vi "RuptureAnalysis.vi"(10 "Tracenames":string[](array[string])) -> ()   [LabVIEW 2018]
uses:
  <vilib>/Utility/file.llb/Read From Spreadsheet File (string).vi
  <vilib>/Utility/file.llb/Write To Spreadsheet File (string).vi
  <vilib>/Analysis/NI_AALPro.lvlib
panel:
  out "Fit result":string[][](array[string])
  in  "stop":bool
  out "Rupture analysis":cluster{dbl[], "Best Linear Fit":dbl[]}[](graph)
  out "Distribution":dynamicdata(graph) caption="Histogram"
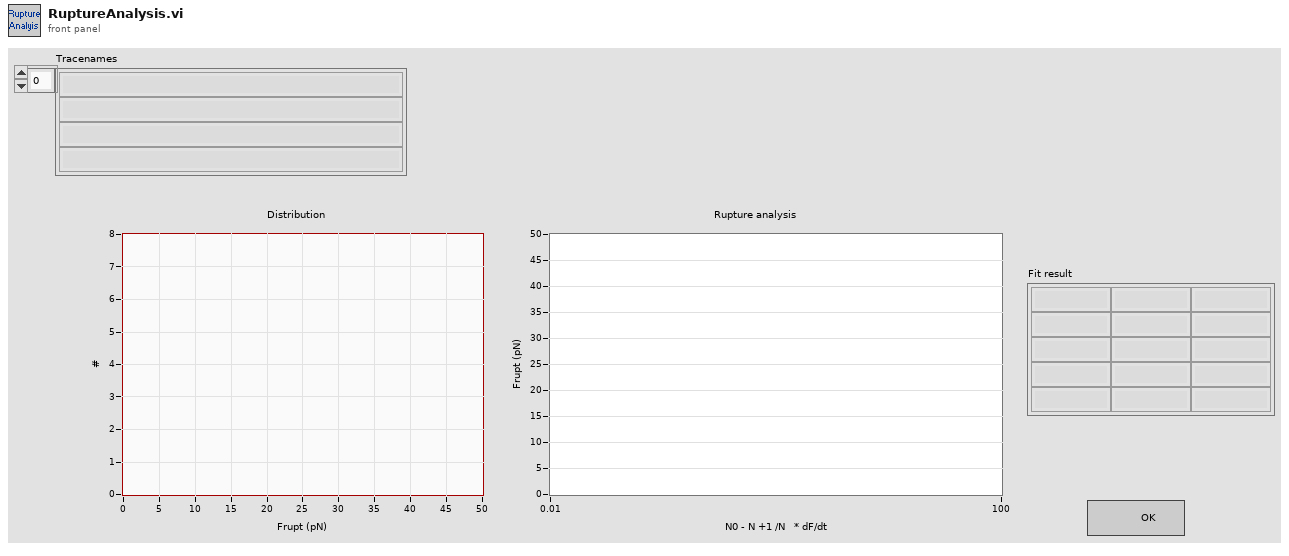
[diagram p1: front panel]
types:
  T1 = enum16{"Init", "Reset", "Update var pars", "Update SE's", "Get", "Save to file", "Read from file"}
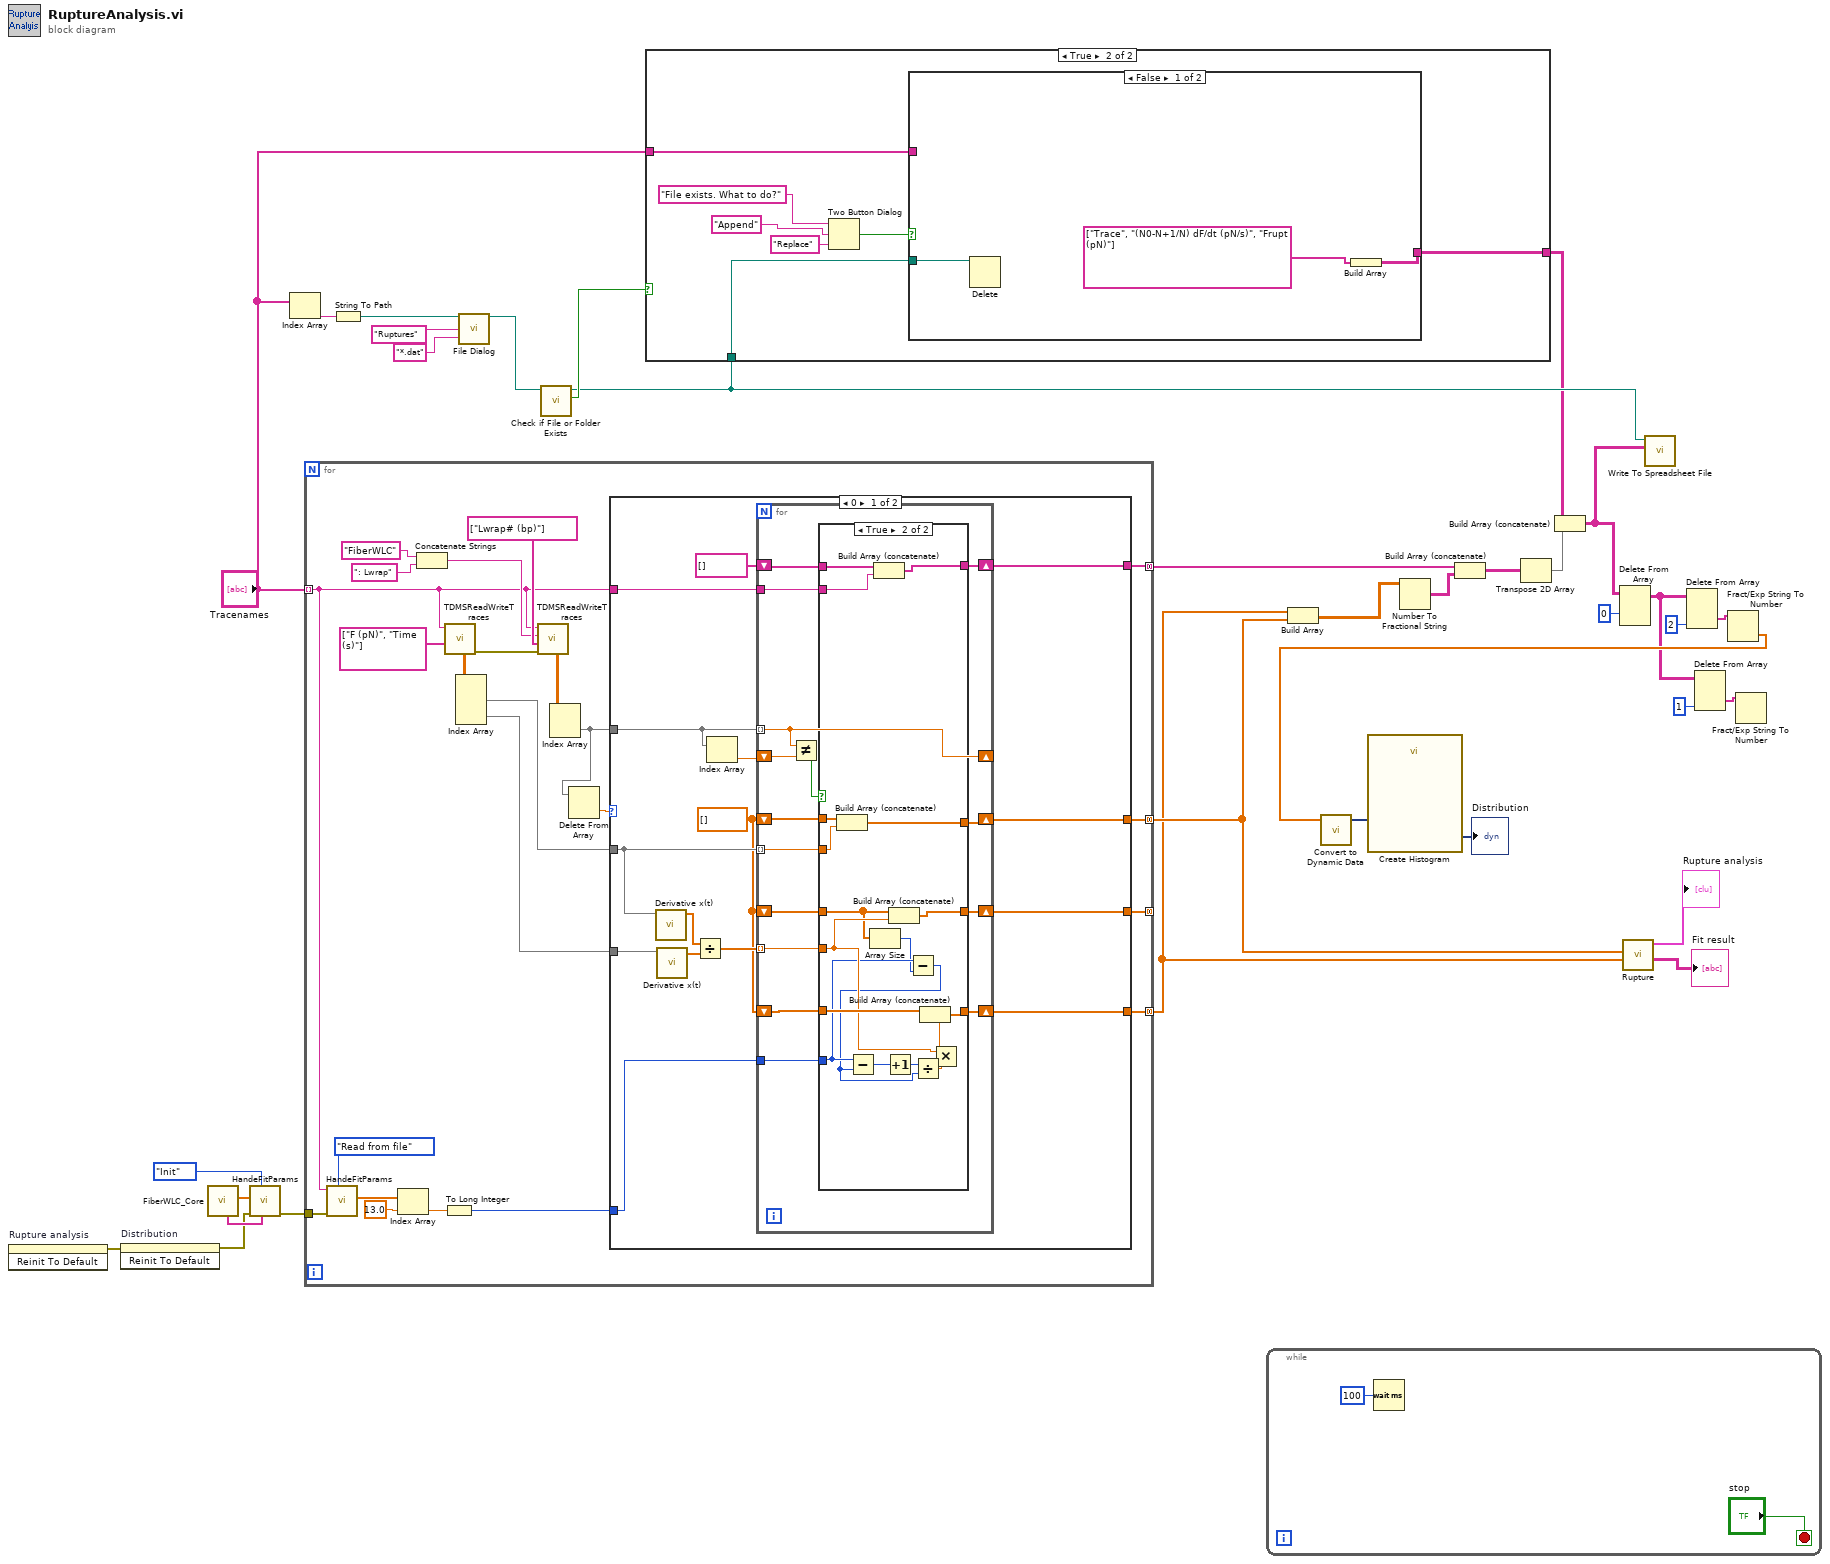
[diagram p0: block diagram]
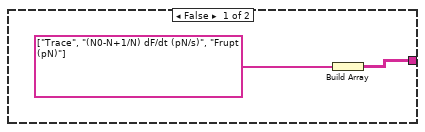
[diagram p2: hidden frame]
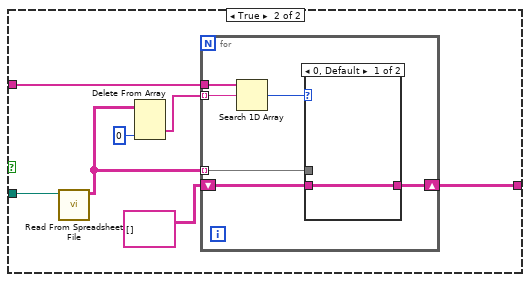
[diagram p3: hidden frame]
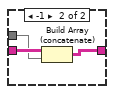
[diagram p4: hidden frame]
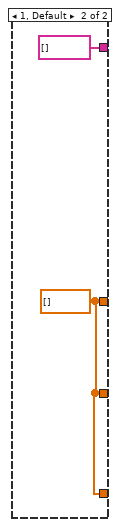
[diagram p6: hidden frame]
diagram:
  n1 = invoke on="Rupture analysis" class="XYGraph (strict)" method="Reinit To Default"() -> (error out=w6:errorcluster)  [unwired: 3 in, 2 out]
  n2 = invoke on="Distribution" class="WFGraph (strict)" method="Reinit To Default"(error in=w6) -> (error out=w7:errorcluster)  [unwired: 2 in, 2 out]
  n3 = call "FiberWLC_Core.vi"() -> ("default params"=w31:dbl[], "default parnames"=w32:string[])  [unwired: 8 in, 2 out]
  n4 = call "HandeFitParams.vi"("Par names"=w32, "task"=T1."Init", "error in (no error)"=w7, "Vars in"=w31) -> ("error out"=w29:errorcluster)  [unwired: 4 in, 3 out]
  n5 = Index Array(array="Tracenames") -> (element=w21:string)  [unwired: 1 in]
  n6 = for {
    tunnel: "Tracenames" -> [w36] mode=indexing
    tunnel: [w49] -> w4 mode=concatenating
    tunnel: [w46] -> _ mode=concatenating
    tunnel: w29 -> [w40]
    tunnel: [w38] -> w3 mode=concatenating
    tunnel: [w35] -> w22 mode=concatenating
    n7 = call "HandeFitParams.vi"("task"=T1."Read from file", "error in (no error)"=w40, "tracename in"=w36) -> ("Vars out"=w42:dbl[])  [unwired: 5 in, 3 out]
    n8 = Index Array(array=w42, index=13.0 ("element")) -> (element=w39:dbl)
    n9 = Concatenate Strings("FiberWLC" ("group name"), ": Lwrap" ("string")) -> (w56:string)
    n10 = To Long Integer(number=w39) -> (32bit integer=w37:i32)
    n11 = call "TDMSReadWriteTraces.vi"("Channels in"=string[] ["F (pN)", "Time (s)"] ("channel name(s) in"), "tracename"=w36) -> ("error out"=w52:errorcluster, "Data out"=w50:dbl[][])  [unwired: 4 in, 4 out]
    n12 = Index Array(array=w50) -> (element #1=w48:dbl[], element #2=w47:dbl[])  [unwired: 4 in]
    n13 = call "TDMSReadWriteTraces.vi"("error in (no error)"=w52, "Channels in"=string[] ["Lwrap# (bp)"], "group name"=w56, "tracename"=w36) -> ("Data out"=w53:dbl[][])  [unwired: 2 in, 5 out]
    n14 = Index Array(array=w53) -> (element=w45:dbl[])  [unwired: 2 in]
    n15 = Delete From Array(array=w45) -> (deleted portion=w44:dbl)  [unwired: 2 in, 1 out]
    n16 = case shown="0" w44 {
      tunnel: [w71 w111] -> w49
      tunnel: w48 -> [w65 _]
      tunnel: w47 -> [w70 _]
      tunnel: [w66 w111] -> w46
      tunnel: w45 -> [w64 _]
      tunnel: w37 -> [w63 _]
      tunnel: [w61 w111] -> w38
      tunnel: w36 -> [w60 _]
      tunnel: [w59 string[] []] -> w35
      frame 0 {
        w62 = dbl[] []
        n17 = call <vilib>:"Derivative x(t).vi"("X"=w65) -> ("dX/dt"=w69:dbl[])  [unwired: 9 in, 1 out]
        n18 = call <vilib>:"Derivative x(t).vi"("X"=w70) -> ("dX/dt"=w68:dbl[])  [unwired: 9 in, 1 out]
        n19 = Divide(x=w69, y=w68) -> (x/y=w67:dbl[])
        n20 = Index Array(array=w64) -> (element=w72:dbl)  [unwired: 1 in]
        n21 = for {
          shift-right: [w86] -> _
          shift-left: w72 -> [w87]
          tunnel: w64 -> [w86] mode=indexing
          tunnel: w65 -> [w83] mode=indexing
          shift-right: [w82] -> w71
          shift-left: w62 -> [w84]
          shift-right: [w81] -> w66
          shift-left: w62 -> [w80]
          tunnel: w67 -> [w79] mode=indexing
          tunnel: w63 -> [w78]
          shift-right: [w77] -> w61
          shift-left: w62 -> [w76]
          shift-right: [w73] -> w59
          shift-left: string[] [] -> [w74]
          tunnel: w60 -> [w75]
          n22 = Not Equal?(x=w86, y=w87) -> (x != y?=w85:bool)
          n23 = case shown="True" w85 {
            tunnel: w84 -> [w91 w109]
            tunnel: w83 -> [_ w108]
            tunnel: [w91 w107] -> w82
            tunnel: [w90 w106] -> w81
            tunnel: w80 -> [w90 w96]
            tunnel: w79 -> [_ w99]
            tunnel: w78 -> [_ w98]
            tunnel: [w89 w103] -> w77
            tunnel: w76 -> [w89 w102]
            tunnel: w75 -> [_ w94]
            tunnel: w74 -> [w88 w93]
            tunnel: [w88 w92] -> w73
            frame False {
            }
            frame True {
              n24 = Build Array (concatenate)(w109, w108) -> (w107:dbl[])
              n25 = Array Size(array=w96) -> (size(s)=w97:i32)
              n26 = Build Array (concatenate)(w93, w94) -> (w92:string[])
              n27 = Build Array (concatenate)(w96, w99) -> (w106:dbl[])
              n28 = Subtract(x=w98, y=w97) -> (x-y=w95:i32)
              n29 = Subtract(x=w98, y=w95) -> (x-y=w105:i32)
              n30 = Increment(x=w105) -> (x+1=w104:i32)
              n31 = Divide(x=w104, y=w95) -> (x/y=w101:dbl)
              n32 = Multiply(x=w99, y=w101) -> (x*y=w100:dbl)
              n33 = Build Array (concatenate)(w102, w100) -> (w103:dbl[])
            }
          }
        }
      }
      frame 1, Default {
        w111 = dbl[] []
      }
    }
  }
  n34 = String To Path(string=w21) -> (path=w20:path)
  n35 = call "File Dialog"("start path"=w20, "default name"="Ruptures", "pattern (all files)"="*.dat") -> ("selected path"=w19:path)  [unwired: 9 in, 3 out]
  n36 = call <vilib>:"Check if File or Folder Exists.vi"("path"=w19) -> ("file or folder exists?"=w18:bool, "dup path"=w17:path)  [unwired: 8 in, 1 out]
  n37 = case shown="True" w18 {
    tunnel: w17 -> [_ w116]
    tunnel: [w112 w115] -> w16
    tunnel: "Tracenames" -> [_ w114]
    frame False {
      n38 = Build Array(string[] ["Trace", "(N0-N+1/N) dF/dt (pN/s)", "Frupt (pN)"]) -> (w112:string[][])
    }
    frame True {
      n39 = Two Button Dialog(message="File exists. What to do?", 1:"Replace" ("F button name (\"Cancel\")"), 2:"Append" ("T button name (\"OK\")")) -> (T button?=w117:bool)
      n40 = case shown="False" w117 {
        tunnel: w116 -> [w123 w130]
        tunnel: [w121 w124] -> w115
        tunnel: w114 -> [_ w127]
        frame False {
          n41 = Delete(path (use dialog)=w123) -> ()  [unwired: 4 in, 3 out]
          n42 = Build Array(string[] ["Trace", "(N0-N+1/N) dF/dt (pN/s)", "Frupt (pN)"]) -> (w121:string[][])
        }
        frame True {
          n43 = call-poly <vilib>:"Read From Spreadsheet File.vi"("file path (dialog if empty)"=w130) -> ("all rows"=w126:string[][])  [unwired: 6 in, 4 out]
          n44 = Delete From Array(array=w126, index (col)=0 ("disabled index (col)")) -> (deleted portion=w128:string[])  [unwired: 2 in, 1 out]
          n45 = for {
            tunnel: w128 -> [w136] mode=indexing
            tunnel: w127 -> [w135]
            shift-right: [w131] -> w124
            shift-left: string[][] [] ("all rows") -> [w133]
            tunnel: w126 -> [w132] mode=indexing
            n46 = Search 1D Array(1D array=w135, element=w136) -> (index of element=w134:i32)  [unwired: 1 in]
            n47 = case shown="0, Default" w134 {
              tunnel: w133 -> [w137 w140]
              tunnel: [w137 w139] -> w131
              tunnel: w132 -> [_ w138]
              frame 0, Default {
              }
              frame -1 {
                n48 = Build Array (concatenate)(w140, w138) -> (w139:string[][])
              }
            }
          }
        }
      }
    }
  }
  n49 = while {
    stop <- "stop" stop-if-true
    n50 = Wait (ms)(milliseconds to wait=u32 100) -> ()  [unwired: 1 out]
  }
  n51 = Build Array(w3, w4) -> (w28:dbl[][])
  n52 = Number To Fractional String(number=w28) -> (F-format string=w27:string[][])  [unwired: 3 in]
  n53 = Build Array (concatenate)(w22, w27) -> (w26:string[][])
  n54 = Transpose 2D Array(2D array=w26) -> (transposed array=w25:string[][])
  n55 = Build Array (concatenate)(w16, w25) -> (w15:string[][])
  n56 = Delete From Array(array=w15, index (row)=0) -> (array with subset deleted=w8:string[][])  [unwired: 2 in, 1 out]
  n57 = call "Rupture.vi"("(N0-N+1/N) dF/dt (pN/s)"=w3, "Frupt (pN)"=w4) -> ("Fit result"=→"Fit result":string[][], "Rupture analysis"=→"Rupture analysis":cluster{dbl[], "Best Linear Fit":dbl[]}[])  [unwired: 7 in, 1 out]
  n58 = call-poly <vilib>:"Write To Spreadsheet File.vi"("2D data"=w15, "file path (dialog if empty)"=w17) -> ()  [unwired: 6 in, 1 out]
  n59 = Delete From Array(array=w8, index (col)=2 ("disabled index (col)")) -> (deleted portion=w12:string[])  [unwired: 2 in, 1 out]
  n60 = Delete From Array(array=w8, index (col)=1 ("disabled index (col)")) -> (deleted portion=w10:string[])  [unwired: 2 in, 1 out]
  n61 = Fract/Exp String To Number(string=w12) -> (number=w11:dbl[])  [unwired: 3 in, 1 out]
  n62 = call "Convert to Dynamic Data"("Array"=w11) -> ("Dynamic Data Type"=w34:dynamicdata)  [unwired: 3 in]
  n63 = call "Create Histogram"("Signal"=w34) -> ("Histogram"=→"Distribution":dynamicdata)  [unwired: 9 in, 1 out]
  n64 = Fract/Exp String To Number(string=w10) -> ()  [unwired: 3 in, 2 out]
